vi "new_navigator.vi"(10 "velocity from motor Controllor (m/s)":dbl, 11 "x acceleration (g)":dbl) -> ()   [LabVIEW 2018]
uses:
  <vilib>/Analysis/NI_AALPro.lvlib
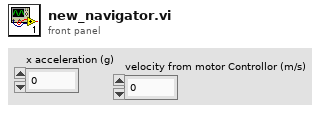
[diagram p1: front panel]
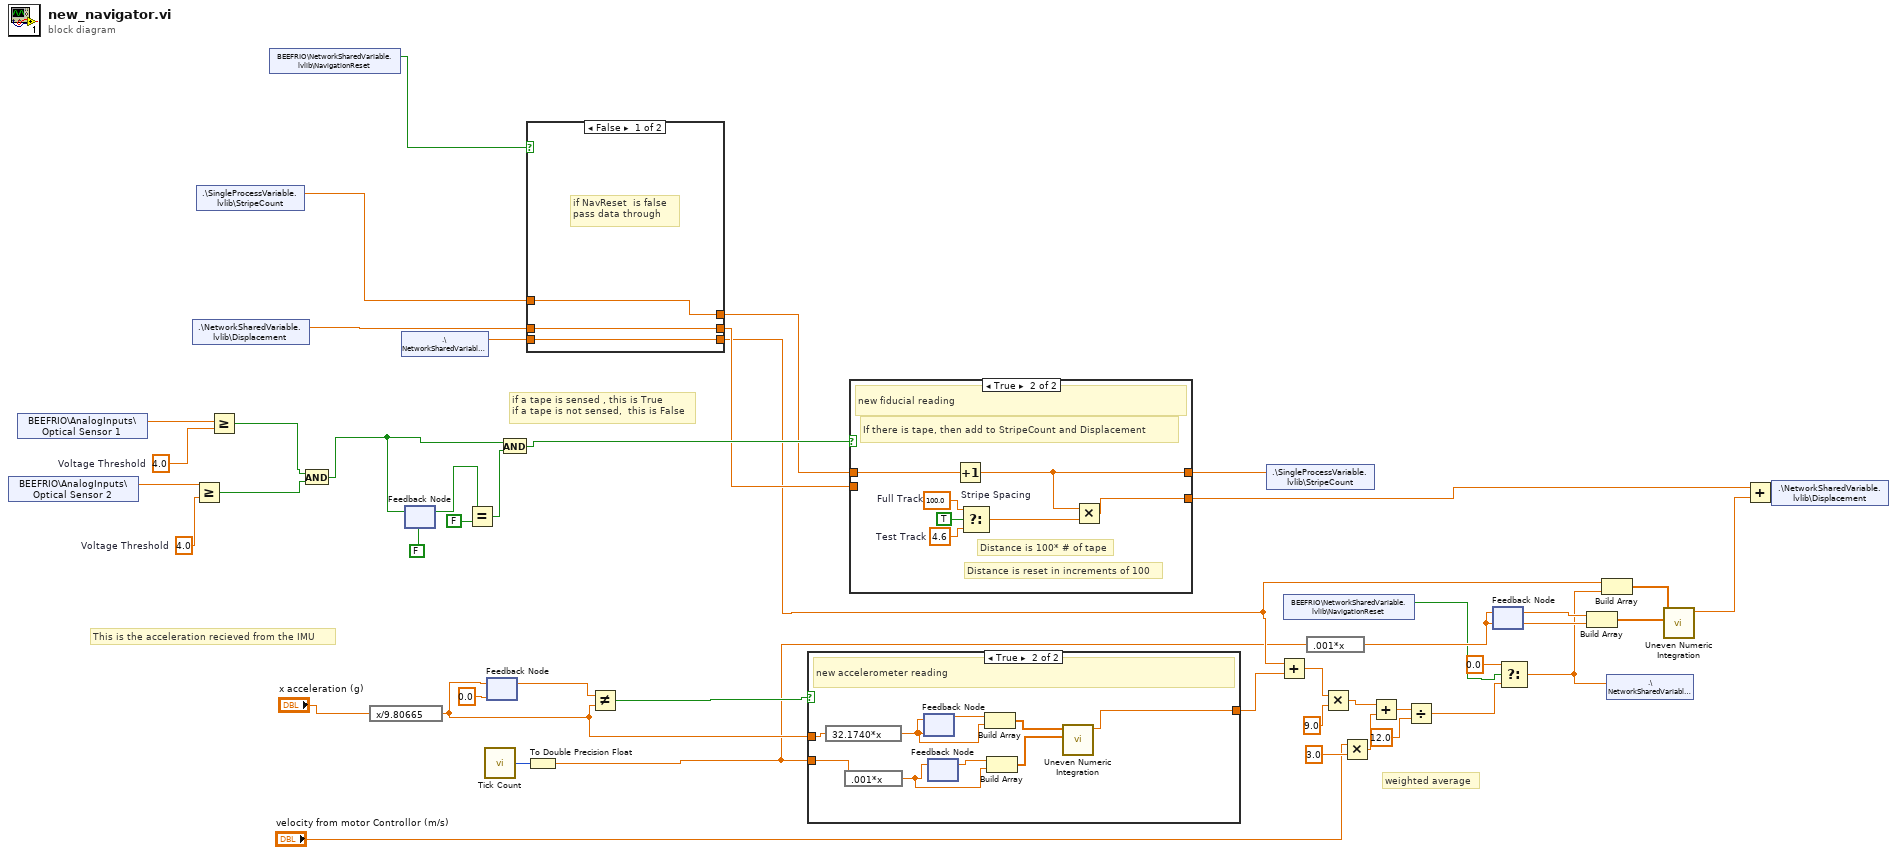
[diagram p0: block diagram]
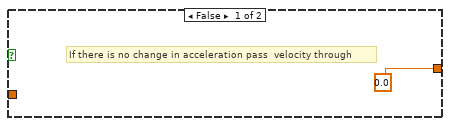
[diagram p2: hidden frame]
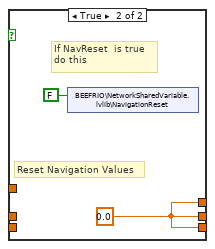
[diagram p3: hidden frame]
diagram:
  w42 = 4.0  # Voltage Threshold
  w47 = 4.0  # Voltage Threshold
  # "weighted average"
  # "This is the acceleration recieved from the IMU"
  # "if a tape is sensed , this is True\nif a tape is not sensed,  this is False"
  n1 = shared-variable "BEEFRIO\\AnalogInputs\\Optical Sensor 2"() -> (w41:dbl)  [unwired: 1 in, 1 out]
  n2 = shared-variable "BEEFRIO\\AnalogInputs\\Optical Sensor 1"() -> (w29:dbl)  [unwired: 1 in, 1 out]
  n3 = shared-variable ".\\NetworkSharedVariable.lvlib\\Displacement"() -> (w34:dbl)  [unwired: 1 in, 1 out]
  n4 = Greater Or Equal?(x=w41, y=w42) -> (x >= y?=w39:bool)
  n5 = shared-variable ".\\SingleProcessVariable.lvlib\\StripeCount"() -> (w35:dbl)  [unwired: 1 in, 1 out]
  n6 = Greater Or Equal?(x=w29, y=w47) -> (x >= y?=w40:bool)
  n7 = shared-variable "BEEFRIO\\NetworkSharedVariable.lvlib\\NavigationReset"() -> (w33:bool)  [unwired: 1 in, 1 out]
  n8 = And(x=w40, y=w39) -> (x .and. y?=w38:bool)
  n9 = expression code="x/9.80665"("x acceleration (g)") -> (w24:dbl)
  n10 = shared-variable ".\\NetworkSharedVariable.lvlib\\Velocity"() -> (w36:dbl)  [unwired: 1 in, 1 out]
  n11 = feedback #1(FALSE) -> (w43:bool)
  n12 = feedback-in #1(w38) -> ()
  n13 = Equal?(x=w43, y=FALSE) -> (x = y?=w44:bool)
  n14 = call "Tick Count"() -> ("Tick Count(mSec)"=w25:u32)
  n15 = feedback #2(0.0 ("x acceleration (g)")) -> (w26:dbl)
  n16 = feedback-in #2(w24) -> ()
  n17 = And(x=w38, y=w44) -> (x .and. y?=w37:bool)
  n18 = case shown="False" w33 {
    tunnel: w35 -> [w50 _]
    tunnel: [w50 w51] -> w32
    tunnel: [w49 w51] -> w31
    tunnel: w34 -> [w49 _]
    tunnel: w36 -> [w48 _]
    tunnel: [w48 w51] -> w13
    frame False {
      # "if NavReset  is false\npass data through"
    }
    frame True {
      w51 = 0.0
      # "Reset Navigation Values"
      # "If NavReset  is true\ndo this"
      n19 = shared-variable "BEEFRIO\\NetworkSharedVariable.lvlib\\NavigationReset"(FALSE ("NavReset")) -> ()  [unwired: 1 in, 1 out]
    }
  }
  n20 = To Double Precision Float(number=w25) -> (double precision float=w9:dbl)
  n21 = Not Equal?(x=w26, y=w24) -> (x != y?=w17:bool)
  n22 = case shown="True" w17 {
    tunnel: w24 -> [_ w62]
    tunnel: w9 -> [_ w58]
    tunnel: [0.0 ("0") w54] -> w4
    frame False {
      # "If there is no change in acceleration pass  velocity through"
    }
    frame True {
      # "new accelerometer reading"
      n23 = expression code="32.1740*x"(w62) -> (w59:dbl)
      n24 = expression code=".001*x"(w58) -> (w56:dbl)
      n25 = feedback #3(w59) -> (w61:dbl)
      n26 = feedback-in #3(w59) -> ()
      n27 = feedback #4() -> (w57:dbl)  [unwired: 1 in]
      n28 = feedback-in #4(w56) -> ()
      n29 = Build Array(w61, w59) -> (w60:dbl[])
      n30 = Build Array(w57, w56) -> (w55:dbl[])
      n31 = call <vilib>:"Uneven Numeric Integration.vi"("T"=w55, "X"=w60) -> ("result"=w54:dbl)  [unwired: 8 in, 1 out]
    }
  }
  n32 = case shown="True" w37 {
    tunnel: [w64 w69] -> w30
    tunnel: w32 -> [w64 w71]
    tunnel: [w63 w70] -> w15
    tunnel: w31 -> [w63 _]
    frame False {
      # "If there is no new tape pass value through"
    }
    frame True {
      w68 = 4.6  # Test Track
      w67 = 100.0  # Full Track
      # "Distance is reset in increments of 100"
      # "Distance is 100* # of tape"
      # "If there is tape, then add to StripeCount and Displacement"
      # "new fiducial reading"
      n33 = Increment(x=w71) -> (x+1=w69:dbl)
      n34 = Select "Stripe Spacing"(t=w67, s=TRUE, f=w68) -> (s? t:f=w66:dbl)
      n35 = Multiply(x=w69, y=w66) -> (x*y=w70:dbl)
    }
  }
  n36 = shared-variable ".\\SingleProcessVariable.lvlib\\StripeCount"(w30) -> ()  [unwired: 1 in, 1 out]
  n37 = Add(x=w13, y=w4) -> (x+y=w2:dbl)
  n38 = shared-variable "BEEFRIO\\NetworkSharedVariable.lvlib\\NavigationReset"() -> (w6:bool)  [unwired: 1 in, 1 out]
  n39 = expression code=".001*x"(w9) -> (w11:dbl)
  n40 = Multiply(x=w2, y=9.0) -> (x*y=w22:dbl)
  n41 = Multiply(x="velocity from motor Controllor (m/s)", y=3.0) -> (x*y=w21:dbl)
  n42 = Add(x=w22, y=w21) -> (x+y=w23:dbl)
  n43 = Divide(x=w23, y=12.0) -> (x/y=w3:dbl)
  n44 = feedback #5() -> (w12:dbl)  [unwired: 1 in]
  n45 = feedback-in #5(w11) -> ()
  n46 = Select(t=0.0, s=w6, f=w3) -> (s? t:f=w5:dbl)
  n47 = Build Array(w12, w11) -> (w10:dbl[])
  n48 = Build Array(w13, w5) -> (w14:dbl[])
  n49 = shared-variable ".\\NetworkSharedVariable.lvlib\\Velocity"(w5) -> ()  [unwired: 1 in, 1 out]
  n50 = call <vilib>:"Uneven Numeric Integration.vi"("T"=w10, "X"=w14) -> ("result"=w8:dbl)  [unwired: 8 in, 1 out]
  n51 = Add(x=w15, y=w8) -> (x+y=w16:dbl)
  n52 = shared-variable ".\\NetworkSharedVariable.lvlib\\Displacement"(w16) -> ()  [unwired: 1 in, 1 out]
